vi "Read FunctionIniFilePath.vi"(8 "error in (no error)":errorcluster, 11 "FunctionBase in":refnum<class "FunctionBase.lvclass">) -> (0 "error out":errorcluster, 2 "FunctionIniFilePath":path, 3 "FunctionBase out":refnum<class "FunctionBase.lvclass">)   [LabVIEW 2018, in "Functions.lvlib" / "FunctionBase.lvclass"]
uses:
  FunctionBase.lvclass
  FunctionBase.lvclass/FunctionBase.ctl
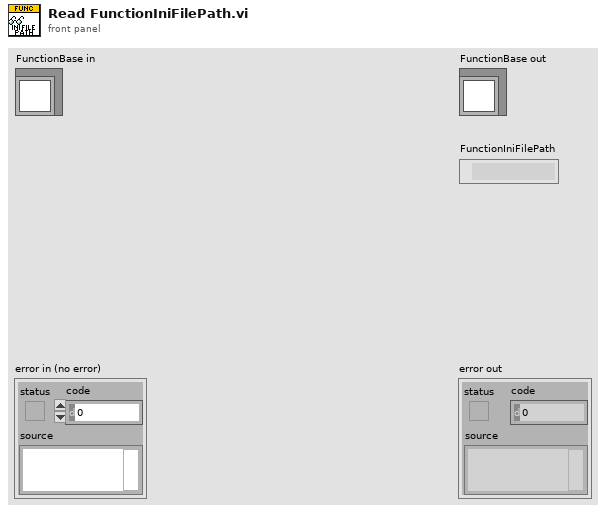
[diagram p1: front panel]
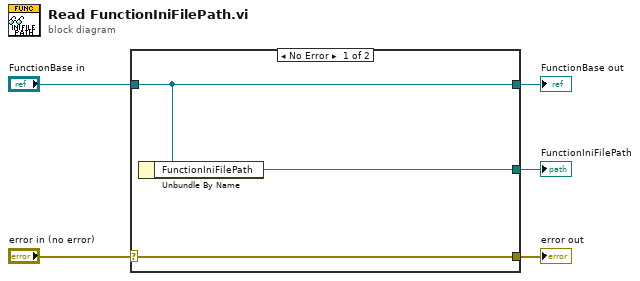
[diagram p0: block diagram]
diagram:
  n1 = case shown="No Error" "error in (no error)" {
    selector: "error in (no error)" -> [w8 w9]
    tunnel: [w8 w9] -> w4
    tunnel: [w7 w10] -> w2
    tunnel: "FunctionBase in" -> [w7 w10]
    tunnel: [w6 _] -> w1
    frame No Error {
      n2 = Unbundle By Name(w7) -> ("FunctionIniFilePath"=w6:path)
    }
    frame Error {
    }
  }
  "error out" <- w4
  "FunctionBase out" <- w2
  "FunctionIniFilePath" <- w1
